vi "StateMachine.vi"() -> ()   [LabVIEW 2014]
uses:
  C:/Users/elg2252/Documents/State Enum.ctl
panel:
  in  "Menu":T1
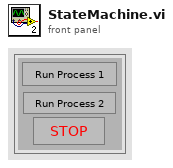
[diagram p1: front panel]
types:
  T1 = cluster{"Process 1":bool, "Process 2":bool, "stop":bool}
  T2 = typedef "State Enum.ctl" = enum32{"Idle", "Process 1", "Process 2", "Stop"}
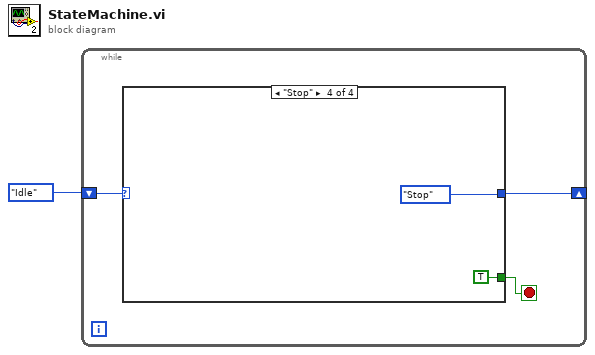
[diagram p0: block diagram]
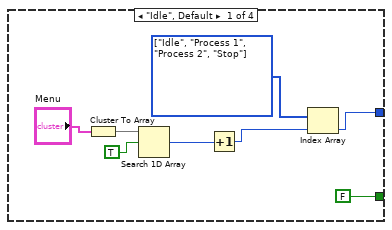
[diagram p2: hidden frame]
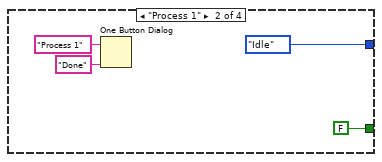
[diagram p3: hidden frame]
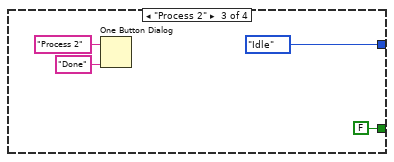
[diagram p4: hidden frame]
diagram:
  n1 = while {
    shift-right: [w2] -> _
    shift-left: State_Enum."Idle" ("State Enum") -> [w4]
    stop <- w3 stop-if-true
    n2 = case shown="\"Stop\"" w4 {
      tunnel: [FALSE FALSE FALSE TRUE] -> w3
      tunnel: [w10 State_Enum."Idle" ("State Enum") State_Enum."Idle" ("State Enum") State_Enum."Stop" ("State Enum")] -> w2
      frame "Idle", Default {
        w11 = T2[] [enum."Idle", enum."Process 1", enum."Process 2", enum."Stop"] items=["Idle", "Process 1", "Process 2", "Stop"]
        n3 = Cluster To Array(cluster="Menu") -> (array=w8:bool[])
        n4 = Search 1D Array(1D array=w8, element=TRUE) -> (index of element=w6:i32)  [unwired: 1 in]
        n5 = Increment(x=w6) -> (x+1=w5:i32)
        n6 = Index Array(array=w11, index=w5) -> (element=w10:T2)
      }
      frame "Process 1" {
        n7 = One Button Dialog(message="Process 1", button name ("OK")="Done") -> ()  [unwired: 1 out]
      }
      frame "Process 2" {
        n8 = One Button Dialog(message="Process 2", button name ("OK")="Done") -> ()  [unwired: 1 out]
      }
      frame "Stop" {
      }
    }
  }
